vi "Fire User Event - Stop.vi"(8 "error in (no error)":T1 caption="Fehler (Eingang, kein Fehler)", 11 "Benutzerereignis - Stopp":refnum<user-event>) -> (0 "error out":T1 caption="Fehler (Ausgang)")   [LabVIEW 2014, in "MyQH User Event - Stop.lvlib"]
doc: "Sendet das Stoppereignis, um die Schleife zur Ereignisbehandlung anzuhalten."
uses:
  MyQH User Event - Stop.lvlib
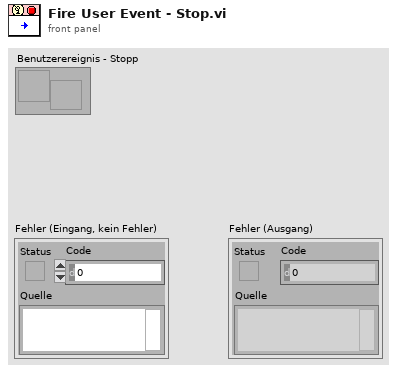
[diagram p1: front panel]
types:
  T1 = cluster{"Status":bool, "Code":i32, "Quelle":string}
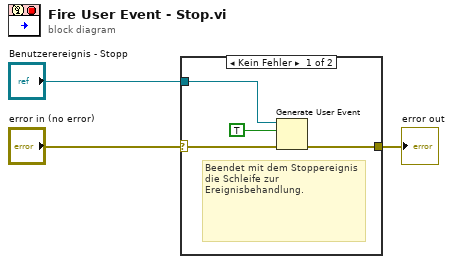
[diagram p0: block diagram]
diagram:
  n1 = case shown="Kein Fehler" "error in (no error)" {
    selector: "error in (no error)" -> [w4 w8]
    tunnel: [w6 w8] -> w3
    tunnel: "Benutzerereignis - Stopp" -> [w5 _]
    frame No Error {
      # "Beendet mit dem Stoppereignis die Schleife zur Ereignisbehandlung."
      n2 = Generate User Event(user event=w5, event data cluster=TRUE ("event data"), error in=w4) -> (error out=w6:errorcluster)  [unwired: 1 in, 1 out]
    }
    frame Error {
    }
  }
  "error out" <- w3
